vi "test_TCP_constants_packet_start.vi"() -> (2 "output_byte":u8=60, 3 "output_char":string="<")   [LabVIEW 2014]
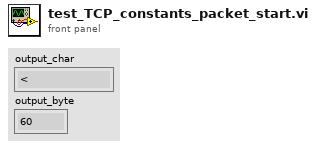
[diagram p1: front panel]
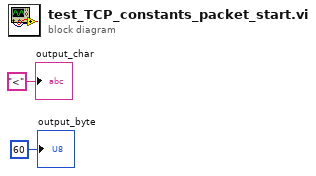
[diagram p0: block diagram]
diagram:
  "output_char" <- "<"
  "output_byte" <- u8 60
